vi "Prime FFT.vi"(0 "X":cdb[](array[numeric]) format="%.2f") -> (1 "FFT {X}":cdb[](array[numeric]) format="%.2f", 2 "error":i32)   [LabVIEW 2017, in "NI_Gmath.lvlib"]
doc: "A special form of the Fourier transform. Use this VI if signal length is a prime."
uses:
  NI_Gmath.lvlib
  Complex FFT.vi
  Inverse Real FFT.vi
  NI_AALPro.lvlib
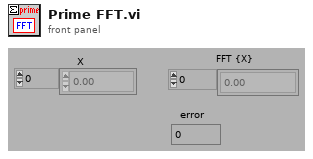
[diagram p1: front panel]
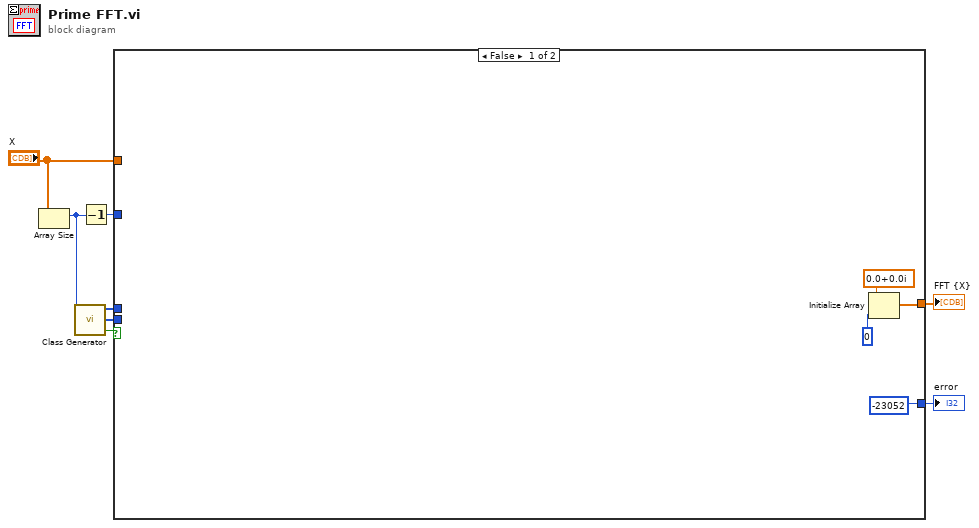
[diagram p0: block diagram]
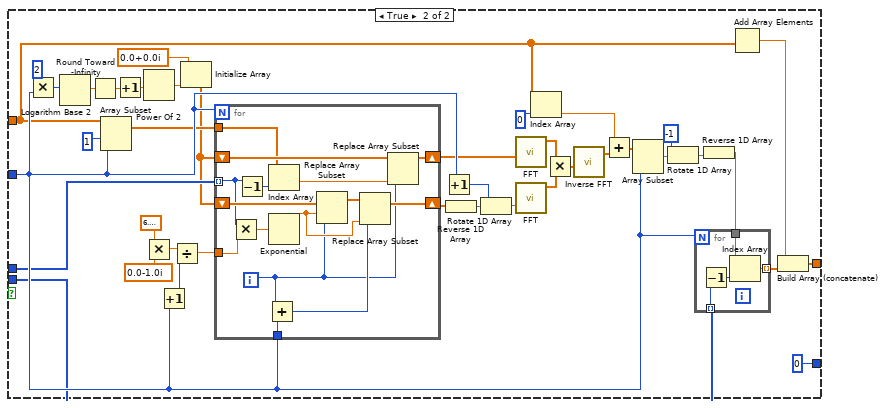
[diagram p2: hidden frame]
diagram:
  n1 = Array Size(array="X") -> (size(s)=w6:i32)
  n2 = call "Class Generator.vi"("#"=w6) -> ("psi"=w8:i32[], "psi^-1"=w7:i32[], "prime"=w1:bool)
  n3 = Decrement(x=w6) -> (x-1=w5:i32)
  n4 = case shown="False" w1 {
    tunnel: "X" -> [_ w13]
    tunnel: w5 -> [_ w45]
    tunnel: w7 -> [_ w44]
    tunnel: w8 -> [_ w43]
    tunnel: [w10 w15] -> w3
    tunnel: [-23052 0] -> w2
    frame False {
      n5 = Initialize Array(cdb 0.0+0.0i, 0) -> (w10:cdb[])
    }
    frame True {
      n6 = Multiply(x=2, y=w45) -> (x*y=w47:i32)
      n7 = Logarithm Base 2(1:w47) -> (0:w48:dbl)
      n8 = Round Toward -Infinity(1:w48) -> (0:w49:dbl)
      n9 = Array Subset(array=w13, index=1, length=w45) -> (w37:cdb[])
      n10 = Increment(x=w49) -> (x+1=w50:dbl)
      n11 = Power Of 2(x=w50) -> (2^x=w51:dbl)
      n12 = Multiply(x=6.283185307179586, y=cdb 0.0-1.0i) -> (x*y=w20:cdb)
      n13 = Increment(x=w45) -> (x+1=w26:i32)
      n14 = Divide(x=w20, y=w26) -> (x/y=w21:cdb)
      n15 = Initialize Array(cdb 0.0+0.0i, w51) -> (w17:cdb[])
      n16 = for {
        N: w45 -> [_]
        shift-right: [w65] -> w36
        shift-left: w17 -> [w66]
        tunnel: w43 -> [w56] mode=indexing
        shift-right: [w59] -> w30
        shift-left: w17 -> [w64]
        tunnel: w21 -> [w63]
        tunnel: w45 -> [w62]
        tunnel: w37 -> [w55]
        i -> [w52]
        n17 = Multiply(x=w56, y=w63) -> (x*y=w53:cdb)
        n18 = Decrement(x=w56) -> (x-1=w57:i32)
        n19 = Add(x=w52, y=w62) -> (x+y=w61:i32)
        n20 = Index Array(array=w55, index=w57) -> (element=w58:cdb)
        n21 = Exponential(1:w53) -> (0:w54:cdb)
        n22 = Replace Array Subset(array=w64, new element=w54, index=w52) -> (w60:cdb[])
        n23 = Replace Array Subset(array=w60, new element=w54, index=w61) -> (w59:cdb[])
        n24 = Replace Array Subset(array=w66, new element=w58, index=w52) -> (w65:cdb[])
      }
      n25 = Increment(x=w45) -> (x+1=w29:i32)
      n26 = Reverse 1D Array(array=w30) -> (reversed array=w22:cdb[])
      n27 = Rotate 1D Array(1:w22, 2:w29) -> (0:w38:cdb[])
      n28 = call-poly "FFT.vi"("X"=w36) -> ("FFT {X}"=w23:cdb[])  [unwired: 9 in, 1 out]
      n29 = call-poly "FFT.vi"("X"=w38) -> ("FFT {X}"=w25:cdb[])  [unwired: 9 in, 1 out]
      n30 = Index Array(array=w13, index=0) -> (element=w39:cdb)
      n31 = Multiply(x=w23, y=w25) -> (x*y=w24:cdb[])
      n32 = call-poly "Inverse FFT.vi"("FFT {X}"=w24) -> ("X"=w40:dbl[])  [unwired: 9 in, 1 out]
      n33 = Add(x=w39, y=w40) -> (x+y=w31:cdb[])
      n34 = Array Subset(array=w31, length=w45) -> (w41:cdb[])  [unwired: 1 in]
      n35 = Rotate 1D Array(1:w41, 2:-1) -> (0:w35:cdb[])
      n36 = Reverse 1D Array(array=w35) -> (reversed array=w42:cdb[])
      n37 = for {
        N: w45 -> [_]
        tunnel: w44 -> [w70] mode=indexing
        tunnel: [w69] -> w33 mode=indexing
        tunnel: w42 -> [w67]
        n38 = Decrement(x=w70) -> (x-1=w68:i32)
        n39 = Index Array(array=w67, index=w68) -> (element=w69:cdb)
      }
      n40 = Add Array Elements(numeric array=w13) -> (sum=w32:cdb)
      n41 = Build Array (concatenate)(w32, w33) -> (w15:cdb[])
    }
  }
  "FFT {X}" <- w3
  "error" <- w2
